vi "Main.vi"() -> ()   [LabVIEW 2021]
uses:
  controls/States.ctl
  <vilib>/MakerHub/LINX/Public/Peripherals/Digital/Digital Read 1 Chan.vi
  <vilib>/MakerHub/LINX/Public/Peripherals/Digital/Digital Read N Chans.vi
  <vilib>/MakerHub/LINX/Private/Local IO/LinxDigitalRead.vi
  <vilib>/MakerHub/LINX/Public/Utilities/Check Channel.vi
  <vilib>/MakerHub/LINX/Public/Utilities/Open Serial.vi
  <vilib>/MakerHub/LINX/Public/Sensors/Motion/Servo/Servo Open One Channel.vi
  <vilib>/MakerHub/LINX/Private/Utilties/Generate Error.vi
  <vilib>/MakerHub/LINX/Public/Peripherals/Analog/Analog Write 1 Chan.vi
  <vilib>/MakerHub/LINX/Public/Sensors/Motion/Servo/Servo Set Pulse Width One Channel.vi
  <vilib>/MakerHub/LINX/Public/Sensors/Motion/Servo/Servo Close One Channel.vi
  <vilib>/vision/NI_Vision_Development_Module.lvlib
  <vilib>/MakerHub/LINX/LMH-LINX.lvlib
  <vilib>/MakerHub/LINX/Public/Sensors/Motion/Servo/Servo.lvlib
panel:
  in  "DC Motor PWM":dbl
  in  "DC Motor Channel":u8
  in  "Servo  PWM":u16
  in  "Servo Channel":u8
  in  "Serial Port":refnum<visa-resource-name>="N/A"
  in  "IR Channel":u8
  out "Error Flag":bool
  in  "Rotation Angle Ranges":cluster{sgl, sgl}[](array[cluster]) {"?" format="%.2f"; "?" format="%.2f"}
  out "Matches":T1(array[cluster]) {"Bounding Box"."y" format="%.2f"; "Bounding Box"."x" format="%.2f"; "Position"."y" format="%.2f"; "Position"."x" format="%.2f"; "Score" format="%.2f"; "Scale" format="%.2f"; "Angle" format="%.2f"}
  in  "Minimum Match Score":sgl=800.0
  in  "Number of Matches Requested":i32=2
  out "Crop Out":T2(plugin-control) caption="Image Out"
  out "Image Out":T2(plugin-control)
  in  "Directory":path
  out "Vision Out":T2(plugin-control) caption="Image Out"
  out "IR Flag":bool
  in  "Take Photo Button":bool
  out "Stop Flag":bool
  in  "Match Button":bool
  in  "Open Button":bool
  in  "Create Pattern Button":bool
  in  "Stop Button":bool caption="Stop"
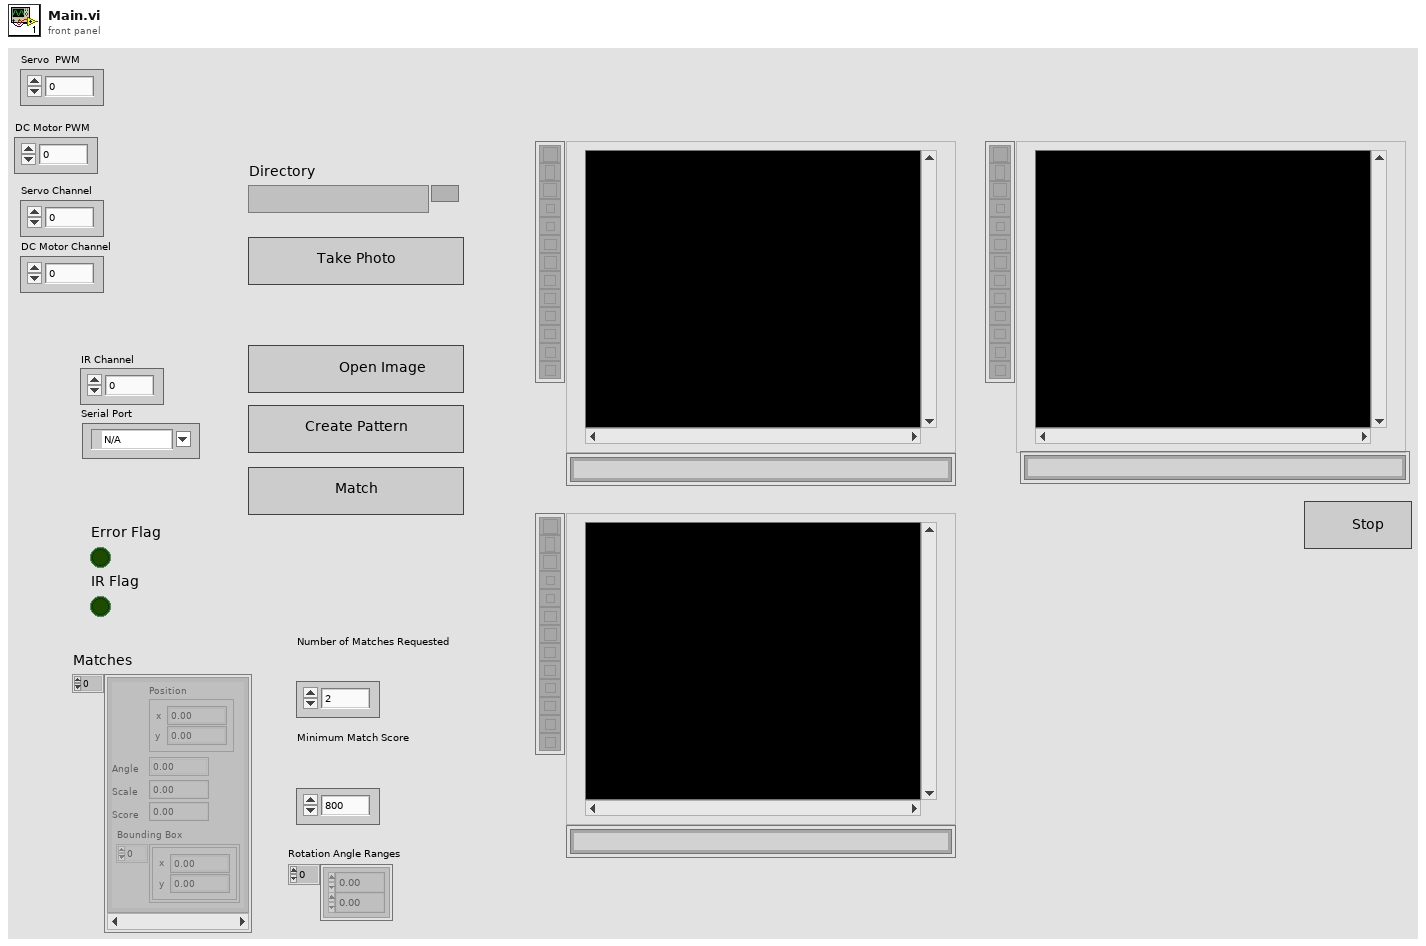
[diagram p1: front panel]
types:
  T1 = cluster{"Position":cluster{"x":sgl, "y":sgl}, "Angle":sgl, "Scale":sgl, "Score":sgl, "Bounding Box":cluster{"x":sgl, "y":sgl}[]}[]
  T2 = typedef "IMAQ Image.ctl" = refnum<image>
  T3 = typedef "States.ctl" = enum16{"INIT", "ACCEPT", "REJECT", "CAPTURE", "CREATE", "MATCH", "OPEN", "STOP"}
  T4 = typedef "LMH-LINX.lvlib/LINX Ref.ctl" = cluster{"IO":T5, "Interface":T6, "LINX Device Config":T7}
  T5 = typedef "LMH-LINX.lvlib/Platform.ctl" = enum16{"Remote", "Local"}
  T6 = typedef "LMH-LINX.lvlib/Interface.ctl" = enum16{"Serial", "TCP"}
  T7 = typedef "LMH-LINX.lvlib/Device.lvlib/LINX Device Config.ctl" = cluster{"Interface":T6, "COM Port":refnum<visa-resource-name>, "TCP Configuration":T8, "Device Family":u8, "Device ID":u8, "Device Name":string, "TCP Ref":refnum<k5>, "Channels":T9}
  T8 = typedef "LMH-LINX.lvlib/Device.lvlib/TCP Config.ctl" = cluster{"IP Address":string, "Port":u16}
  T9 = typedef "LMH-LINX.lvlib/Channels.ctl" = cluster{"DI":u8[], "DO":u8[], "AI":u8[], "AO":u8[], "PWM":u8[], "QE":u8[], "UART":u8[], "I2C 2":u8[], "SPI":u8[], "CAN":u8[], "Servo":u8[], "AI Ref (V)":dbl, "AI Resolution (Bits)":u8, "AO Ref (V)":dbl, "AO Resolution (Bits)":u8}
  T10 = typedef "Image Type" = u32
  T11 = typedef "ROI Descriptor" = cluster{"Global Rectangle":i32[], "Contours":cluster{"ID":enum32{"External", "Internal"}, "Type":u32, "Coordinates":i32[]}[]}
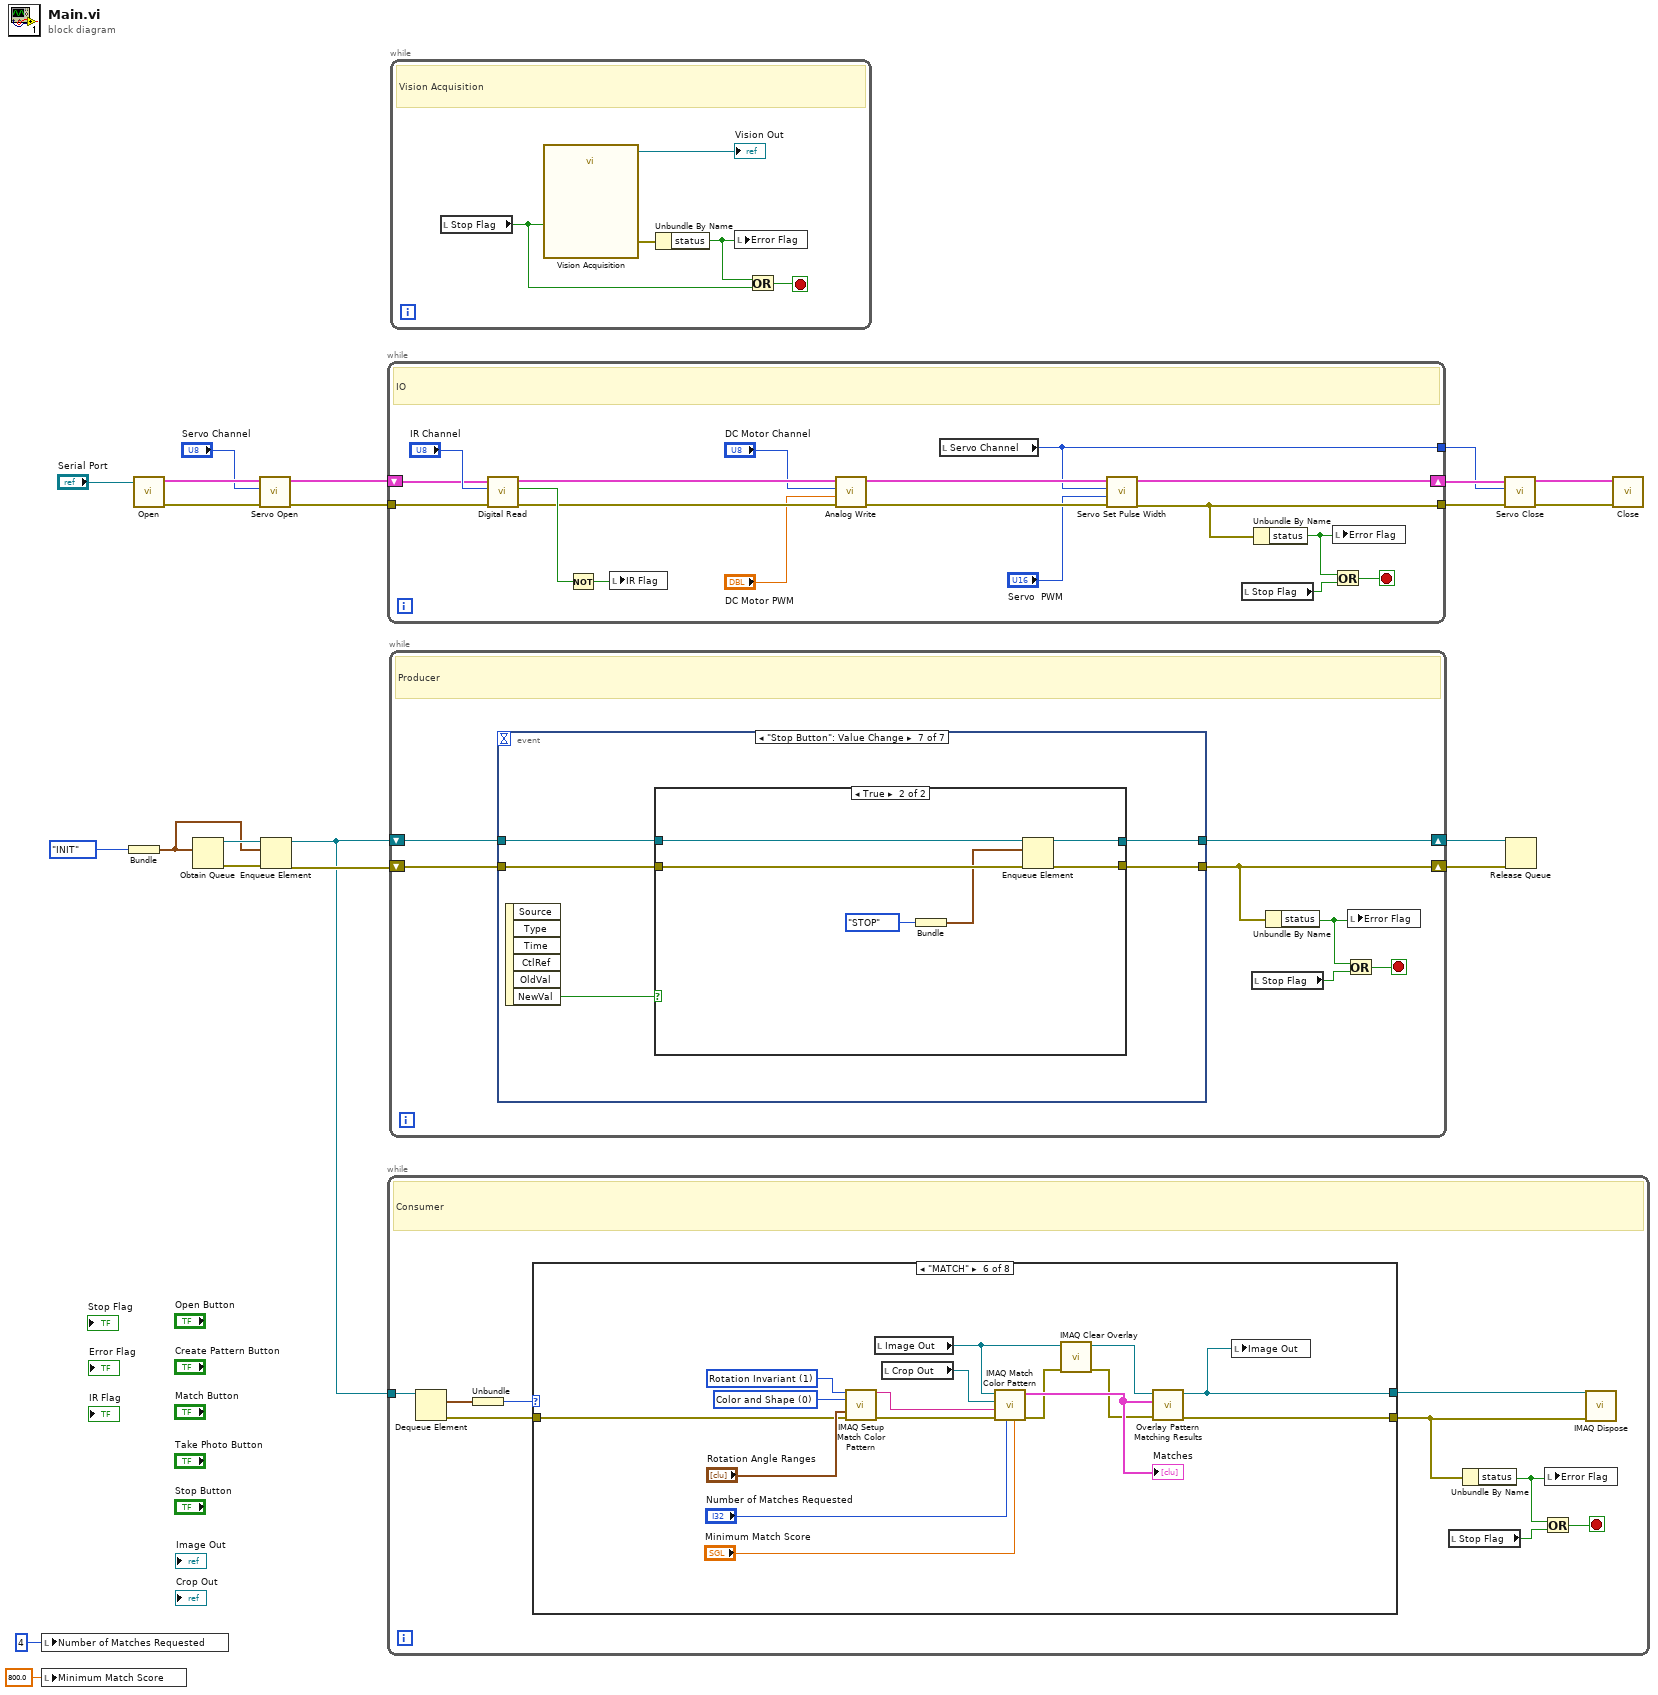
[diagram p0: block diagram]
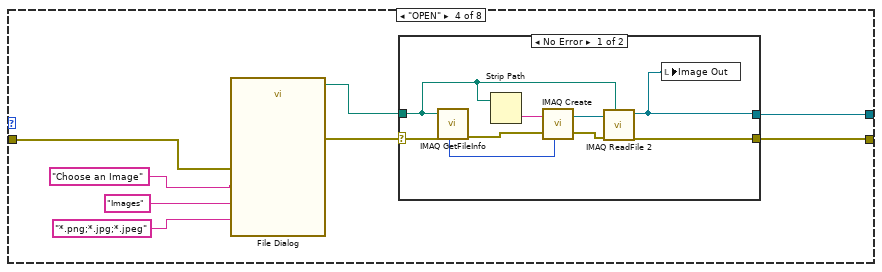
[diagram p5: hidden frame]
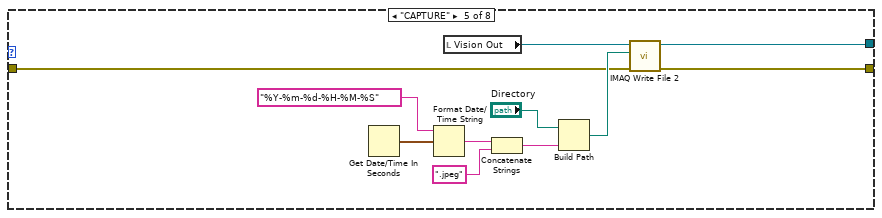
[diagram p7: hidden frame]
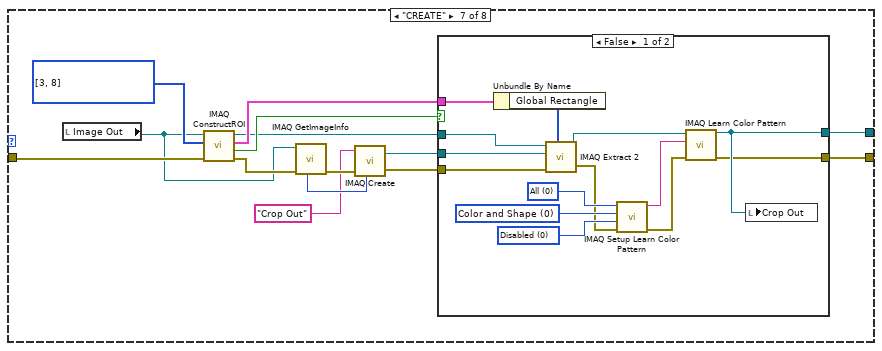
[diagram p8: hidden frame]
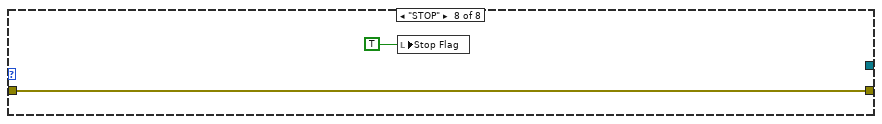
[diagram p10: hidden frame]
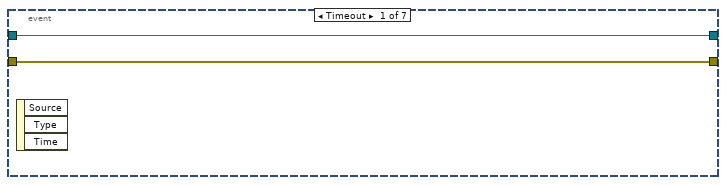
[diagram p11: hidden frame]
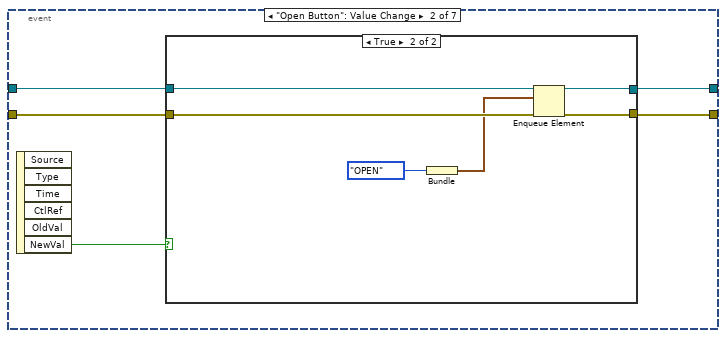
[diagram p12: hidden frame]
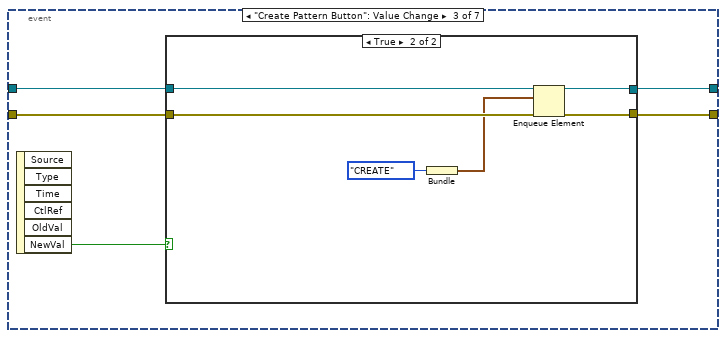
[diagram p14: hidden frame]
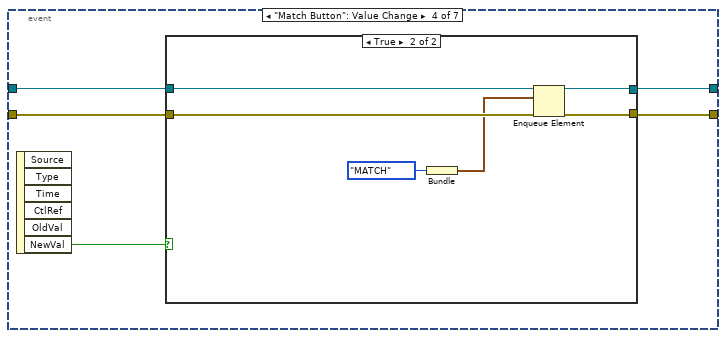
[diagram p16: hidden frame]
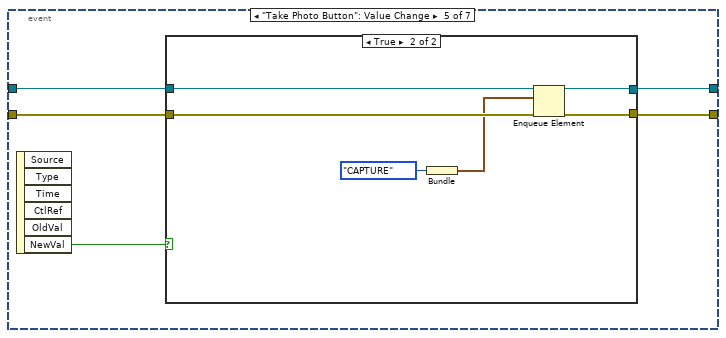
[diagram p18: hidden frame]
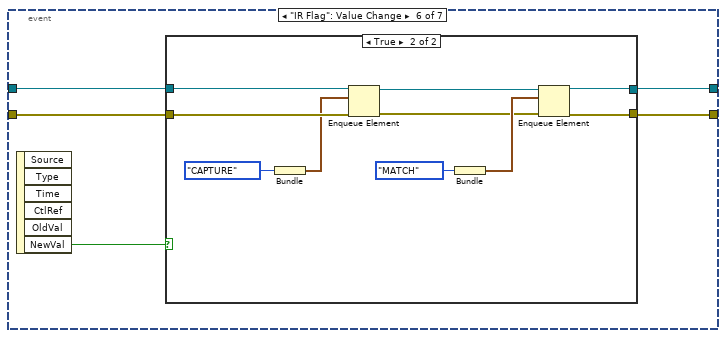
[diagram p20: hidden frame]
diagram:
  n1 = local write "Number of Matches Requested"(4 ("Number of Matches Requested")) -> ()
  n2 = local write "Minimum Match Score"(sgl 800.0 ("Minimum Match Score")) -> ()
  n3 = Bundle(States."INIT") -> (w17:cluster{T3})  [unwired: 1 in]
  n4 = call-poly <vilib>:"Open.vi"("Serial Port"="Serial Port") -> ("Error Out"=w8:errorcluster, "LINX Resource"=w7:T4)  [unwired: 8 in, 1 out]
  n5 = Obtain Queue(element data type=w17) -> (queue out=w18:refnum<queue>, error out=w16:errorcluster)  [unwired: 4 in, 1 out]
  n6 = call-poly <vilib>:"Servo Open.vi"("Error In"=w8, "Servo Channel"="Servo Channel", "LINX Resource"=w7) -> ("Error Out"=w9:errorcluster, "LINX Resource"=w10:T4)  [unwired: 7 in]
  n7 = Enqueue Element(queue=w18, element=w17, error in (no error)=w16) -> (queue out=w12:refnum<queue>, error out=w13:errorcluster)  [unwired: 1 in, 1 out]
  n8 = while {
    tunnel: w9 -> [w37]
    tunnel: [w30] -> w5
    shift-right: [w31] -> w6
    shift-left: w10 -> [w35]
    tunnel: [w22] -> w1
    stop <- w38 stop-if-true
    # "IO"
    n9 = call-poly <vilib>:"Digital Read.vi"("Error In"=w37, "DI Channel"="IR Channel", "LINX Resource"=w35) -> ("Error Out"=w28:errorcluster, "DI Value"=w33:bool, "LINX Resource"=w29:T4)  [unwired: 6 in]
    n10 = Not(x=w33) -> (.not. x?=w34:bool)
    n11 = local write "IR Flag"(w34) -> ()
    n12 = call-poly <vilib>:"Analog Write.vi"("Error In"=w28, "AO Value"="DC Motor PWM", "AO Channel"="DC Motor Channel", "LINX Resource"=w29) -> ("Error Out"=w26:errorcluster, "LINX Resource"=w27:T4)  [unwired: 6 in]
    n13 = local read "Servo Channel"() -> (w22:u8)
    n14 = call-poly <vilib>:"Servo Set Pulse Width.vi"("Error In"=w26, "Pulse Width (uS)"="Servo  PWM", "Servo Channel"=w22, "LINX Resource"=w27) -> ("Error Out"=w30:errorcluster, "LINX Resource"=w31:T4)  [unwired: 6 in]
    n15 = local read "Stop Flag"() -> (w39:bool)
    n16 = Unbundle By Name(w30) -> ("status"=w32:bool)
    n17 = local write "Error Flag"(w32) -> ()
    n18 = Or(x=w32, y=w39) -> (x .or. y?=w38:bool)
  }
  n19 = while {
    tunnel: w12 -> [w47]
    stop <- w43 stop-if-true
    # "Consumer"
    n20 = Dequeue Element(queue=w47) -> (element=w48:cluster{T3}, error out=w45:errorcluster)  [unwired: 2 in, 2 out]
    n21 = Unbundle(w48) -> (w46:T3)
    n22 = case shown="\"MATCH\"" w46 {
      tunnel: w45 -> [w49 w50 w51 w56 w72 w83 w106 w127]
      tunnel: [w49 w50 w51 w58 w71 w82 w99 w127] -> w40
      tunnel: [_ _ _ w59 w70 w81 w100 _] -> w41
      frame "INIT", Default {
      }
      frame "ACCEPT" {
      }
      frame "REJECT" {
      }
      frame "OPEN" {
        n23 = call "File Dialog"("default name"="Choose an Image" ("prompt"), "error in"=w56, "pattern (all files)"="*.png;*.jpg;*.jpeg", "pattern label"="Images") -> ("selected path"=w52:path, "error out"=w57:errorcluster)  [unwired: 8 in, 2 out]
        n24 = case shown="No Error" w57 {
          selector: w57 -> [w62 w69]
          tunnel: [w65 _] -> w59
          tunnel: [w61 w69] -> w58
          tunnel: w52 -> [w60 _]
          frame No Error {
            n25 = call "IMAQ GetFileInfo"("error in (no error)"=w62, "File Path"=w60) -> ("error out"=w64:errorcluster, "Image Type"=w66:T10)  [unwired: 3 in, 5 out]
            n26 = Strip Path(path=w60) -> (name=w67:string)  [unwired: 1 out]
            n27 = call "IMAQ Create"("Image Name"=w67, "Image Type"=w66, "error in (no error)"=w64) -> ("New Image"=w68:T2, "error out"=w63:errorcluster)  [unwired: 2 in]
            n28 = call "IMAQ ReadFile 2"("File Path"=w60, "error in (no error)"=w63, "Image"=w68) -> ("error out"=w61:errorcluster, "Image Out"=w65:T2)  [unwired: 4 in, 3 out]
            n29 = local write "Image Out"(w65) -> ()
          }
          frame Error {
          }
        }
      }
      frame "CAPTURE" {
        n30 = Get Date/Time In Seconds() -> (seconds since 1Jan1904=w76:timestamp)
        n31 = Format Date/Time String(time format string (%c)="%Y-%m-%d-%H-%M-%S", seconds (now)=w76) -> (date/time string=w75:string)  [unwired: 1 in]
        n32 = local read "Vision Out"() -> (w80:T2)
        n33 = Concatenate Strings(w75, ".jpeg" ("string")) -> (w79:string)
        n34 = Build Path(base path="Directory", name or relative path=w79) -> (appended path=w78:path)
        n35 = call-poly "IMAQ Write File 2"("error in (no error)"=w72, "File Path"=w78, "Image"=w80) -> ("error out"=w71:errorcluster, "Image Out (duplicate)"=w70:T2)  [unwired: 7 in]
      }
      frame "MATCH" {
        w87 = u32 0 items=["Color and Shape", "Color", "Shape"] ("Match Feature Mode")
        w88 = u32 1 items=["Shift Invariant", "Rotation Invariant"] ("Match Mode")
        n36 = call "IMAQ Setup Match Color Pattern"("Match Mode"=w88, "Match Feature Mode"=w87, "Rotation Angle Ranges (degrees)"="Rotation Angle Ranges", "error in (no error)"=w83) -> ("Match Color Pattern Setup Data"=w89:string, "error out"=w84:errorcluster)  [unwired: 10 in]
        n37 = local read "Image Out"() -> (w96:T2)
        n38 = local read "Crop Out"() -> (w90:T2)
        n39 = call "IMAQ Match Color Pattern"("Minimum Match Score"="Minimum Match Score", "Number of Matches Requested"="Number of Matches Requested", "error in (no error)"=w84, "Match Color Pattern Setup Data"=w89, "Template Image"=w90, "Image"=w96) -> ("error out"=w86:errorcluster, "Matches"=w93:T1)  [unwired: 3 in, 1 out]
        "Matches" <- w93
        n40 = call "IMAQ Clear Overlay"("error in (no error)"=w86, "Image"=w96) -> ("error out"=w85:errorcluster, "Image Out"=w95:T2)  [unwired: 8 in]
        n41 = call "Overlay Pattern Matching Results.vi"("error in"=w85, "Matches"=w93, "Image"=w95) -> ("error out"=w82:errorcluster, "Image Out"=w81:T2)  [unwired: 7 in]
        n42 = local write "Image Out"(w81) -> ()
      }
      frame "CREATE" {
        w101 = u32[] [3, 8] items=["No Selection", "Point", "Line", "Rectangle", "Oval", "Polygon", "Freehand Region", "Annulus", "Zoom", "Pan", "Broken Line", "Freehand Line", "Rotated Rectangle"] ("Tools")
        n43 = local read "Image Out"() -> (w98:T2)
        n44 = call "IMAQ ConstructROI"("error in (no error)"=w106, "Tools"=w101, "Image"=w98) -> ("error out"=w103:errorcluster, "Cancel"=w110:bool, "ROI Descriptor Out"=w108:T11, "Image Out (duplicate)"=w107:T2)  [unwired: 5 in]
        n45 = call "IMAQ GetImageInfo"("error in (no error)"=w103, "Image"=w98) -> ("error out"=w105:errorcluster, "Image Type"=w104:T10)  [unwired: 2 in, 6 out]
        n46 = call "IMAQ Create"("Image Name"="Crop Out", "Image Type"=w104, "error in (no error)"=w105) -> ("New Image"=w109:T2, "error out"=w102:errorcluster)  [unwired: 2 in]
        n47 = case shown="False" w110 {
          tunnel: w109 -> [w121 w126]
          tunnel: w108 -> [w120 _]
          tunnel: w107 -> [w118 _]
          tunnel: [w115 w126] -> w100
          tunnel: [w112 w125] -> w99
          tunnel: w102 -> [w111 w125]
          frame False {
            w122 = u32 0 items=["Disabled", "Ignore Black", "Ignore White", "Ignore Black and White"] ("Ignore Black and White")
            w123 = u32 0 items=["Color and Shape", "Color", "Shape "] ("Feature Mode")
            w124 = u32 0 items=["All", "Shift Information", "Rotation Information"] ("Learn Mode")
            n48 = Unbundle By Name(w120) -> ("Global Rectangle"=w119:i32[])
            n49 = call "IMAQ Extract 2"("Optional Rectangle"=w119, "error in (no error)"=w111, "Image Dst"=w121, "Image Src"=w118) -> ("error out"=w114:errorcluster, "Image Dst Out"=w117:T2)  [unwired: 6 in]
            n50 = call "IMAQ Setup Learn Color Pattern"("error in (no error)"=w114, "Ignore Black and White"=w122, "Feature Mode"=w123, "Learn Mode"=w124) -> ("error out"=w113:errorcluster, "Learn Color Pattern Setup Data"=w116:string)  [unwired: 6 in]
            n51 = call "IMAQ Learn Color Pattern"("error in (no error)"=w113, "Learn Color Pattern Setup Data"=w116, "Image"=w117) -> ("error out"=w112:errorcluster, "Template Image Out"=w115:T2)  [unwired: 7 in]
            n52 = local write "Crop Out"(w115) -> ()
          }
          frame True {
          }
        }
      }
      frame "STOP" {
        n53 = local write "Stop Flag"(TRUE ("Stop Flag")) -> ()
      }
    }
    n54 = local read "Stop Flag"() -> (w42:bool)
    n55 = Unbundle By Name(w40) -> ("status"=w44:bool)
    n56 = Or(x=w44, y=w42) -> (x .or. y?=w43:bool)
    n57 = local write "Error Flag"(w44) -> ()
    n58 = call "IMAQ Dispose"("Image"=w41, "error in (no error)"=w40) -> ()  [unwired: 4 in, 1 out]
  }
  n59 = while {
    shift-right: [w131] -> w15
    shift-left: w12 -> [w133]
    shift-right: [w130] -> w14
    shift-left: w13 -> [w132]
    stop <- w134 stop-if-true
    # "Producer"
    n60 = event shown="[6] \"Stop Button\": Value Change" {
      selector: _ -> [_ _ _ _ _ _ _]
      dyn-events: _ -> [_ _ _ _ _ _ _]
      timeout: _ -> [_ _ _ _ _ _ _]
      tunnel: w133 -> [w137 w140 w153 w166 w179 w192 w209]
      tunnel: w132 -> [w136 w139 w152 w165 w178 w191 w208]
      tunnel: [w137 w142 w155 w168 w181 w194 w211] -> w131
      tunnel: [w136 w141 w154 w167 w180 w193 w210] -> w130
      event Timeout {
        n61 = event-data() -> ()  [unwired: 1 in, 3 out]
      }
      event "Open Button": Value Change {
        n62 = event-data() -> ("NewVal"=w138:bool)  [unwired: 1 in, 5 out]
        n63 = case shown="True" w138 {
          tunnel: [w144 w150] -> w142
          tunnel: [w143 w149] -> w141
          tunnel: w140 -> [w144 w148]
          tunnel: w139 -> [w143 w147]
          frame False {
          }
          frame True {
            n64 = Bundle(States."OPEN") -> (w145:cluster{T3})  [unwired: 1 in]
            n65 = Enqueue Element(queue=w148, element=w145, error in (no error)=w147) -> (queue out=w150:refnum<queue>, error out=w149:errorcluster)  [unwired: 1 in, 1 out]
          }
        }
      }
      event "Create Pattern Button": Value Change {
        n66 = event-data() -> ("NewVal"=w151:bool)  [unwired: 1 in, 5 out]
        n67 = case shown="True" w151 {
          tunnel: [w157 w163] -> w155
          tunnel: [w156 w162] -> w154
          tunnel: w153 -> [w157 w161]
          tunnel: w152 -> [w156 w160]
          frame False {
          }
          frame True {
            n68 = Bundle(States."CREATE") -> (w158:cluster{T3})  [unwired: 1 in]
            n69 = Enqueue Element(queue=w161, element=w158, error in (no error)=w160) -> (queue out=w163:refnum<queue>, error out=w162:errorcluster)  [unwired: 1 in, 1 out]
          }
        }
      }
      event "Match Button": Value Change {
        n70 = event-data() -> ("NewVal"=w164:bool)  [unwired: 1 in, 5 out]
        n71 = case shown="True" w164 {
          tunnel: [w170 w176] -> w168
          tunnel: [w169 w175] -> w167
          tunnel: w166 -> [w170 w174]
          tunnel: w165 -> [w169 w173]
          frame False {
          }
          frame True {
            n72 = Bundle(States."MATCH") -> (w171:cluster{T3})  [unwired: 1 in]
            n73 = Enqueue Element(queue=w174, element=w171, error in (no error)=w173) -> (queue out=w176:refnum<queue>, error out=w175:errorcluster)  [unwired: 1 in, 1 out]
          }
        }
      }
      event "Take Photo Button": Value Change {
        n74 = event-data() -> ("NewVal"=w177:bool)  [unwired: 1 in, 5 out]
        n75 = case shown="True" w177 {
          tunnel: [w183 w189] -> w181
          tunnel: [w182 w188] -> w180
          tunnel: w179 -> [w183 w187]
          tunnel: w178 -> [w182 w186]
          frame False {
          }
          frame True {
            n76 = Bundle(States."CAPTURE") -> (w184:cluster{T3})  [unwired: 1 in]
            n77 = Enqueue Element(queue=w187, element=w184, error in (no error)=w186) -> (queue out=w189:refnum<queue>, error out=w188:errorcluster)  [unwired: 1 in, 1 out]
          }
        }
      }
      event "IR Flag": Value Change {
        n78 = event-data() -> ("NewVal"=w190:bool)  [unwired: 1 in, 5 out]
        n79 = case shown="True" w190 {
          tunnel: [w196 w199] -> w194
          tunnel: [w195 w197] -> w193
          tunnel: w192 -> [w196 w206]
          tunnel: w191 -> [w195 w205]
          frame False {
          }
          frame True {
            n80 = Bundle(States."CAPTURE") -> (w203:cluster{T3})  [unwired: 1 in]
            n81 = Enqueue Element(queue=w206, element=w203, error in (no error)=w205) -> (queue out=w200:refnum<queue>, error out=w198:errorcluster)  [unwired: 1 in, 1 out]
            n82 = Bundle(States."MATCH") -> (w202:cluster{T3})  [unwired: 1 in]
            n83 = Enqueue Element(queue=w200, element=w202, error in (no error)=w198) -> (queue out=w199:refnum<queue>, error out=w197:errorcluster)  [unwired: 1 in, 1 out]
          }
        }
      }
      event "Stop Button": Value Change {
        n84 = event-data() -> ("NewVal"=w207:bool)  [unwired: 1 in, 5 out]
        n85 = case shown="True" w207 {
          tunnel: [w213 w219] -> w211
          tunnel: [w212 w218] -> w210
          tunnel: w209 -> [w213 w217]
          tunnel: w208 -> [w212 w216]
          frame False {
          }
          frame True {
            n86 = Bundle(States."STOP") -> (w214:cluster{T3})  [unwired: 1 in]
            n87 = Enqueue Element(queue=w217, element=w214, error in (no error)=w216) -> (queue out=w219:refnum<queue>, error out=w218:errorcluster)  [unwired: 1 in, 1 out]
          }
        }
      }
    }
    n88 = local read "Stop Flag"() -> (w135:bool)
    n89 = Unbundle By Name(w130) -> ("status"=w129:bool)
    n90 = Or(x=w129, y=w135) -> (x .or. y?=w134:bool)
    n91 = local write "Error Flag"(w129) -> ()
  }
  n92 = while {
    stop <- w222 stop-if-true
    # "Vision Acquisition"
    n93 = local read "Stop Flag"() -> (w220:bool)
    n94 = call "Vision Acquisition"("Stop (F)"=w220) -> ("Image Out"=→"Vision Out":T2, "error out"=w223:errorcluster)  [unwired: 24 in, 1 out]
    n95 = Unbundle By Name(w223) -> ("status"=w221:bool)
    n96 = local write "Error Flag"(w221) -> ()
    n97 = Or(x=w221, y=w220) -> (x .or. y?=w222:bool)
  }
  n98 = call-poly <vilib>:"Servo Close.vi"("Error In"=w5, "Servo Channel"=w1, "LINX Resource"=w6) -> ("Error Out"=w3:errorcluster, "LINX Resource"=w4:T4)  [unwired: 7 in]
  n99 = Release Queue(queue=w15, error in (no error)=w14) -> ()  [unwired: 1 in, 3 out]
  n100 = call <vilib>:"Close.vi"("Error In"=w3, "LINX Resource"=w4) -> ()  [unwired: 9 in, 1 out]
